vi "Revision Query.vi"(8 "error in (no error)":errorcluster, 11 "VISA resource name":refnum<visa-resource-name>) -> (0 "error out":errorcluster, 1 "Instrument Firmware Revision":string, 2 "Instrument Driver Revision":string, 3 "VISA resource name out":refnum<visa-resource-name>)   [LabVIEW 2019, in "BK Precision 8500B Series.lvlib"]
doc: "Queries the current instrument firmware revision and instrument driver revision.\n\nRefer to the Readme file for detailed driver information including modification history."
uses:
  <instrlib>/BK Precision 8500B Series/BK Precision 8500B Series.lvlib
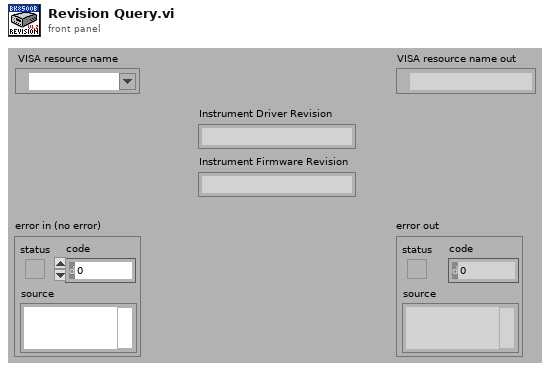
[diagram p1: front panel]
types:
  T1 = cluster{"Major":u16, "Minor":u16, "Fix":u16, "Build":u16}
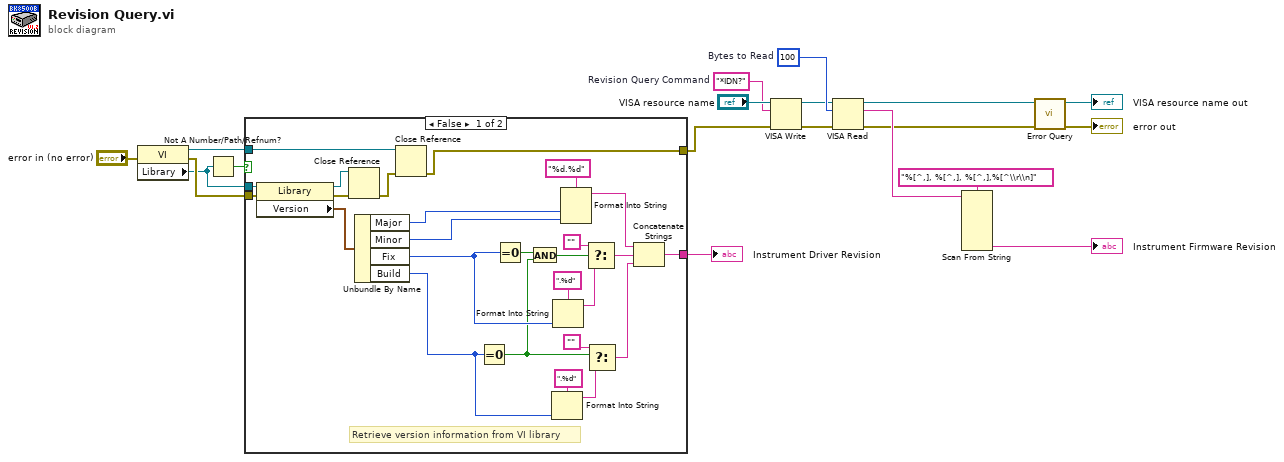
[diagram p0: block diagram]
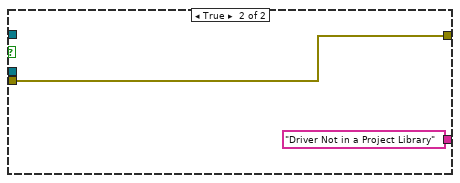
[diagram p2: hidden frame]
diagram:
  w14 = "*IDN?"  # Revision Query Command
  w17 = u32 100  # Bytes to Read
  n1 = property class="VI"(error in="error in (no error)") -> (reference out=w4:refnum<vi>, error out=w3:errorcluster, "Library"=w2:refnum<vi>)  [unwired: 1 in]
  n2 = Not A Number/Path/Refnum?(number/path/refnum=w2) -> (NaN/Path/Refnum?=w1:bool)
  n3 = case shown="False" w1 {
    tunnel: w4 -> [w42 _]
    tunnel: w3 -> [w27 w47]
    tunnel: [w22 w47] -> w5
    tunnel: [w21 "Driver Not in a Project Library"] -> w7
    tunnel: w2 -> [w20 _]
    frame False {
      # "Retrieve version information from VI library"
      n4 = property class="Library"(reference=w20, error in=w27) -> (reference out=w44:refnum<vi>, error out=w45:errorcluster, "Version"=w41:T1)
      n5 = Close Reference(reference=w44, error in (no error)=w45) -> (error out=w43:errorcluster)
      n6 = Unbundle By Name(w41) -> ("Major"=w30:u16, "Minor"=w29:u16, "Fix"=w26:u16, "Build"=w28:u16)
      n7 = Close Reference(reference=w42, error in (no error)=w43) -> (error out=w22:errorcluster)
      n8 = Equal To 0?(x=w28) -> (x = 0?=w24:bool)
      n9 = Equal To 0?(x=w26) -> (x = 0?=w25:bool)
      n10 = And(x=w25, y=w24) -> (x .and. y?=w23:bool)
      n11 = Format Into String(format string=".%d", w28) -> (resulting string=w34:string)  [unwired: 2 in, 1 out]
      n12 = Format Into String(format string=".%d", w26) -> (resulting string=w38:string)  [unwired: 2 in, 1 out]
      n13 = Format Into String(format string="%d.%d", w30, w29) -> (resulting string=w36:string)  [unwired: 2 in, 1 out]
      n14 = Select(t="", s=w23, f=w38) -> (s? t:f=w35:string)
      n15 = Select(t="", s=w24, f=w34) -> (s? t:f=w31:string)
      n16 = Concatenate Strings(w36, w35, w31) -> (w21:string)
    }
    frame True {
    }
  }
  "Instrument Driver Revision" <- w7
  n17 = VISA Write(VISA resource name="VISA resource name", write buffer=w14, error in (no error)=w5) -> (VISA resource name out=w16:refnum<visa-resource-name>, error out=w15:errorcluster)  [unwired: 1 out]
  n18 = VISA Read(VISA resource name=w16, byte count=w17, error in (no error)=w15) -> (VISA resource name out=w10:refnum<visa-resource-name>, read buffer=w13:string, error out=w11:errorcluster)  [unwired: 1 out]
  n19 = Scan From String(format string="%[^,], %[^,], %[^,],%[^\\r\\n]", input string=w13) -> (output 4=→"Instrument Firmware Revision":string)  [unwired: 9 in, 3 out]
  n20 = call <instrlib>:"Error Query.vi"("error in (no error)"=w11, "VISA resource name"=w10) -> ("error out"=→"error out":errorcluster, "VISA resource name out"=→"VISA resource name out":refnum<visa-resource-name>)  [unwired: 6 in, 2 out]
